vi "Compute tau_phi & tau_m from Phasor (Discrete, Ungated).vi"(8 "Error In":errorcluster, 9 "Phasor UCN[W] Parameters":T1, 11 "Phasor":cluster{"X":dbl, "Y":dbl}) -> (0 "Error Out":errorcluster, 1 "Modulus Lifetime":dbl[unit], 3 "Phase Lifetime":dbl[unit])   [LabVIEW 2019]
uses:
  Phasor UC_N[W] Parameters.ctl
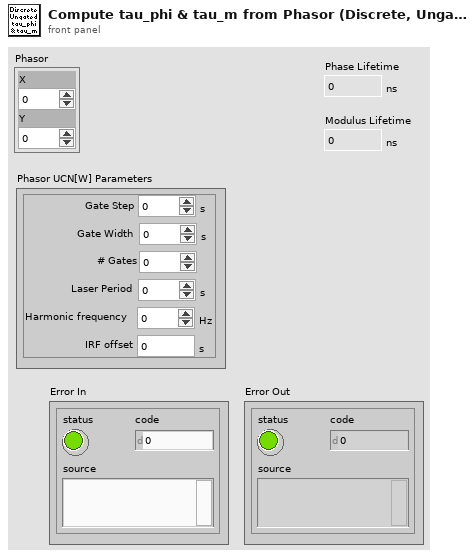
[diagram p1: front panel]
types:
  T1 = typedef "Phasor UC_N[W] Parameters.ctl" = cluster{"Laser Period":dbl[unit], "Gate Width":dbl[unit], "Gate Step":dbl[unit], "Harmonic frequency":dbl[unit], "IRF offset":dbl[unit], "# Gates":dbl}
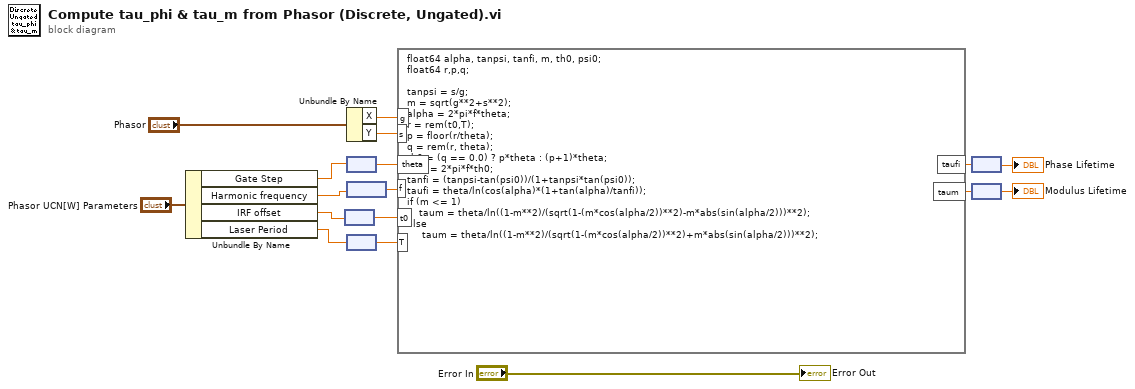
[diagram p0: block diagram]
diagram:
  n1 = Unbundle By Name("Phasor UCN[W] Parameters") -> ("Gate Step"=w5:dbl[unit], "Harmonic frequency"=w4:dbl[unit], "IRF offset"=w3:dbl[unit], "Laser Period"=w2:dbl[unit])
  n2 = node(w3) -> (w8:dbl)
  n3 = Unbundle By Name("Phasor") -> ("X"=w14:dbl, "Y"=w13:dbl)
  n4 = node(w5) -> (w12:dbl)
  n5 = node(w4) -> (w11:dbl)
  n6 = node(w2) -> (w7:dbl)
  n7 = formula code="float64 alpha, tanpsi, tanfi, m, th0, psi0;\nfloat64 r,p,q;\n\ntanpsi = s/g;\nm = sqrt(g**2+s**2);\nalpha = 2*pi*f*theta;\nr = rem(t0,T);\np = floor(r/theta);\nq = rem(r, theta);\nth0 = (q == 0.0) ? p*theta : (p+1)*theta;\npsi0 = 2*pi*f*th0;\ntanfi = (tanpsi-tan(psi0))/(1+tanpsi*tan(psi0));\ntaufi = theta/ln(cos(alpha)*(1+tan(alpha)/tanfi));\nif (m <= 1)\n    taum = theta/ln((1-m**2)/(sqrt(1-(m*cos(alpha/2))**2)-m*abs(sin(alpha/2)))**2);\nelse\n     taum = theta/ln((1-m**2)/(sqrt(1-(m*cos(alpha/2))**2)+m*abs(sin(alpha/2)))**2);"("g"=w14, "s"=w13, "theta"=w12, "f"=w11, "t0"=w8, "T"=w7) -> ("taufi"=w10:dbl, "taum"=w9:dbl)
  n8 = node(w10) -> (→"Phase Lifetime":dbl[unit])
  n9 = node(w9) -> (→"Modulus Lifetime":dbl[unit])
  "Error Out" <- "Error In"
